vi "Manipulator Controller.vi"   [LabVIEW 2018]
uses:
  <vilib>/Rock Robotics/WPI/Joystick/WPI_JoystickDeviceEnum.ctl
  Manipulator Controller Global.vi
types:
  T1 = typedef "WPI_JoystickDeviceEnum.ctl" = enum16{"USB 0", "USB 1", "USB 2", "USB 3", "USB 4", "USB 5"}
  T2 = typedef "WPI_JoystickDevRef.ctl" = cluster{"Device":T1}
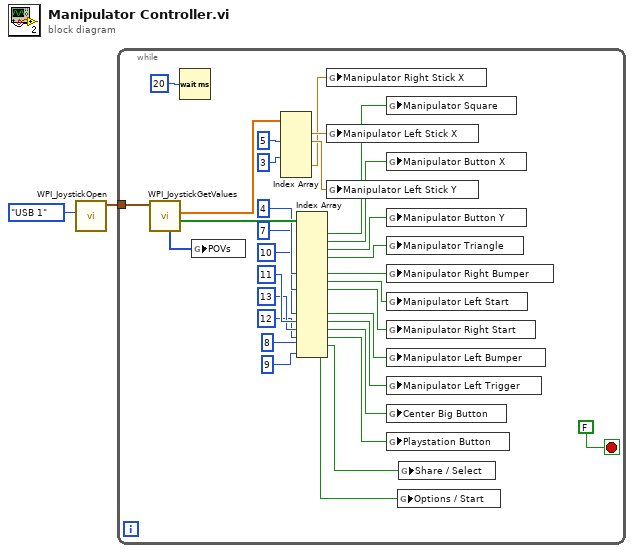
[diagram p0: block diagram]
diagram:
  n1 = call <vilib>:"WPI_JoystickOpen.vi"("JoystickDevice"=WPI_JoystickDeviceEnum."USB 1") -> ("JoystickDevRef"=w1:T2)  [unwired: 10 in]
  n2 = while {
    tunnel: w1 -> [w34]
    stop <- FALSE stop-if-true
    n3 = call <vilib>:"WPI_JoystickGetValues.vi"("JoystickDevRef"=w34) -> ("Buttons"=w32:bool[], "Axes"=w33:dbl[], "POVs"=w16:i16[])  [unwired: 6 in, 2 out]
    n4 = Wait (ms)(milliseconds to wait=u32 20) -> ()  [unwired: 1 out]
    n5 = global write "Manipulator Controller Global.vi" "POVs"(w16) -> ()
    n6 = Index Array(array=w33, index #2=5 ("index"), index #4=3 ("index")) -> (element #1=w31:dbl, element #2=w30:dbl, element #5=w29:dbl)  [unwired: 4 in, 3 out]
    n7 = Index Array(array=w32, index #6=4 ("index"), index #8=7 ("index"), index #11=10 ("index"), index #12=11 ("index"), index #13=13 ("index"), index #14=12 ("index"), index #15=8 ("index"), index #16=9 ("index")) -> (element #1=w28:bool, element #2=w27:bool, element #3=w26:bool, element #4=w15:bool, element #6=w25:bool, element #7=w24:bool, element #8=w23:bool, element #11=w13:bool, element #12=w11:bool, element #13=w9:bool, element #14=w7:bool, element #15=w4:bool, element #16=w3:bool)  [unwired: 8 in, 3 out]
    n8 = global write "Manipulator Controller Global.vi" "Manipulator Right Stick X"(w29) -> ()
    n9 = global write "Manipulator Controller Global.vi" "Manipulator Left Stick X"(w31) -> ()
    n10 = global write "Manipulator Controller Global.vi" "Manipulator Left Stick Y"(w30) -> ()
    n11 = global write "Manipulator Controller Global.vi" "Manipulator Square"(w28) -> ()
    n12 = global write "Manipulator Controller Global.vi" "Manipulator Button X"(w27) -> ()
    n13 = global write "Manipulator Controller Global.vi" "Manipulator Button Y"(w26) -> ()
    n14 = global write "Manipulator Controller Global.vi" "Manipulator Triangle"(w15) -> ()
    n15 = global write "Manipulator Controller Global.vi" "Manipulator Right Bumper"(w25) -> ()
    n16 = global write "Manipulator Controller Global.vi" "Manipulator Left Start"(w24) -> ()
    n17 = global write "Manipulator Controller Global.vi" "Manipulator Right Start"(w23) -> ()
    n18 = global write "Manipulator Controller Global.vi" "Manipulator Left Bumper"(w13) -> ()
    n19 = global write "Manipulator Controller Global.vi" "Manipulator Left Trigger"(w11) -> ()
    n20 = global write "Manipulator Controller Global.vi" "Center Big Button"(w9) -> ()
    n21 = global write "Manipulator Controller Global.vi" "Playstation Button"(w7) -> ()
    n22 = global write "Manipulator Controller Global.vi" "Options / Start"(w3) -> ()
    n23 = global write "Manipulator Controller Global.vi" "Share / Select"(w4) -> ()
  }
